vi "10. FGV Error handler.vi"(5 "error in (no error)":errorcluster) -> (14 "Error message":string="ERROR NO IDENTIFICADO", 15 "Error code":i32)   [LabVIEW 2014]
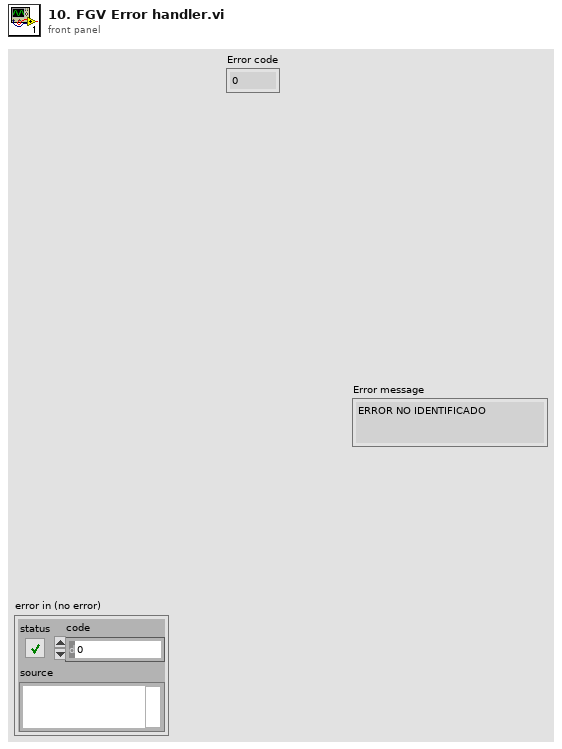
[diagram p1: front panel]
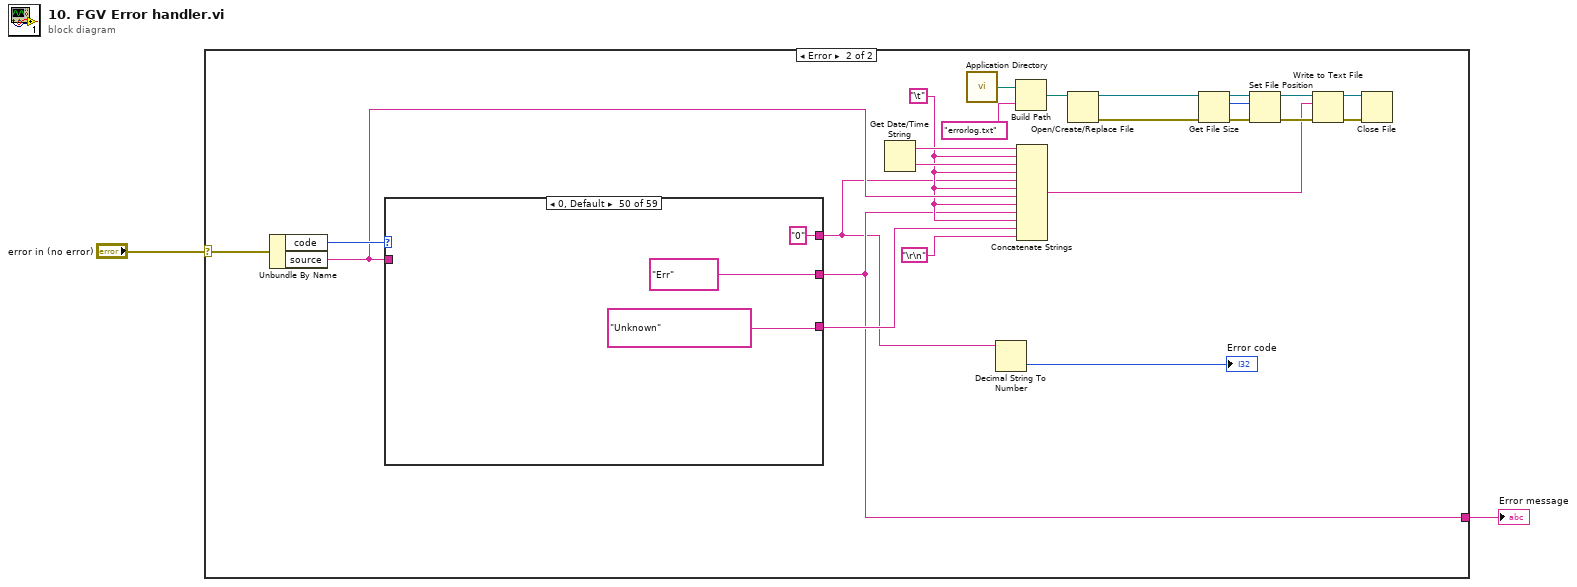
[diagram p0: block diagram]
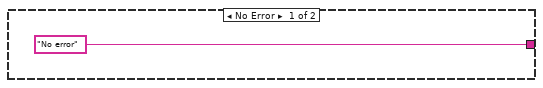
[diagram p2: hidden frame]
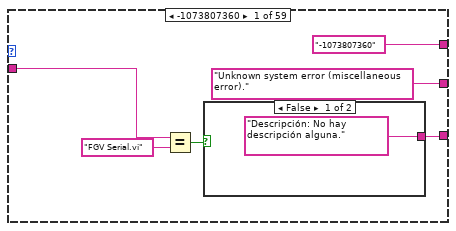
[diagram p3: hidden frame]
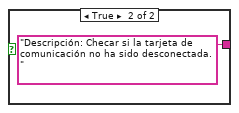
[diagram p4: hidden frame]
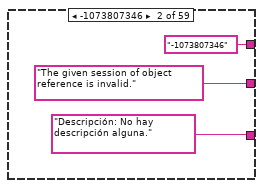
[diagram p5: hidden frame]
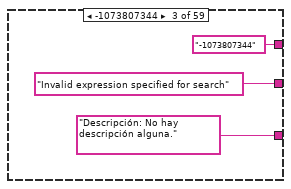
[diagram p6: hidden frame]
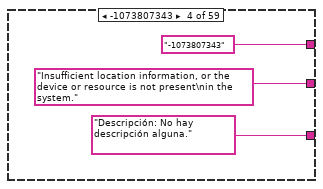
[diagram p7: hidden frame]
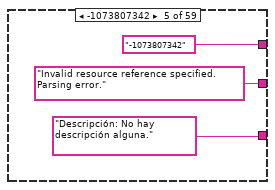
[diagram p8: hidden frame]
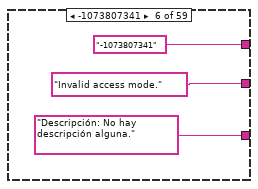
[diagram p9: hidden frame]
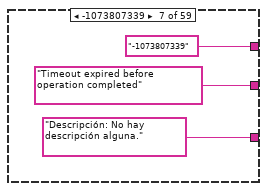
[diagram p10: hidden frame]
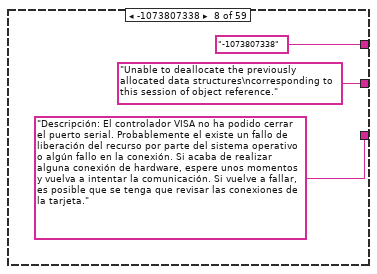
[diagram p11: hidden frame]
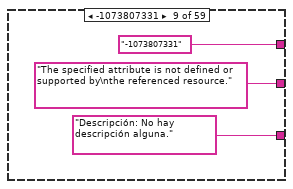
[diagram p12: hidden frame]
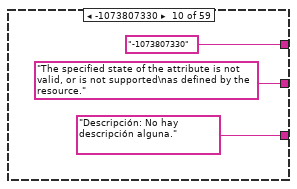
[diagram p13: hidden frame]
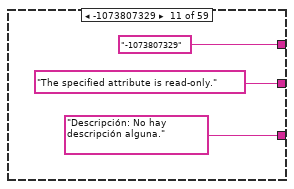
[diagram p14: hidden frame]
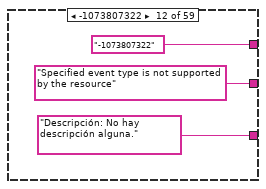
[diagram p15: hidden frame]
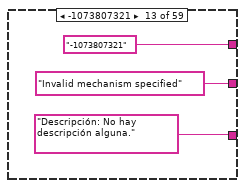
[diagram p16: hidden frame]
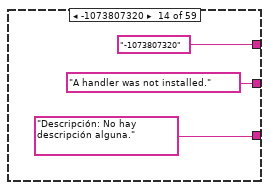
[diagram p17: hidden frame]
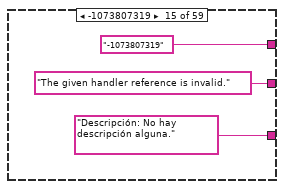
[diagram p18: hidden frame]
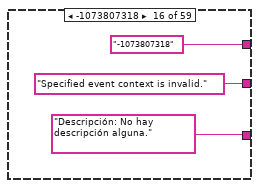
[diagram p19: hidden frame]
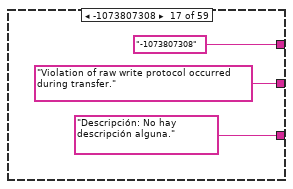
[diagram p20: hidden frame]
diagram:
  n1 = case shown="Error" "error in (no error)" {
    selector: "error in (no error)" -> [_ w26]
    tunnel: ["No error" w6] -> w1
    frame No Error {
    }
    frame Error {
      w9 = "\t"
      n2 = Unbundle By Name(w26) -> ("code"=w27:i32, "source"=w10:string)
      n3 = case shown="0, Default" w27 {
        tunnel: w10 -> [w29 _ _ _ _ _ _ _ _ _ _ _ _ _ _ _ _ _ _ _ _ _ _ _ _ _ _ _ _ _ _ _ _ _ _ _ _ _ _ _ _ _ _ _ _ _ _ _ _ _ _ _ _ _ _ _ _ _ _]
        tunnel: ["Unknown system error (miscellaneous error)." "The given session of object reference is invalid." "Invalid expression specified for search" "Insufficient location information, or the device or resource is not present\nin the system." "Invalid resource reference specified. Parsing error." "Invalid access mode." "Timeout expired before operation completed" "Unable to deallocate the previously allocated data structures\ncorresponding to this session of object reference." "The specified attribute is not defined or supported by\nthe referenced resource." "The specified state of the attribute is not valid, or is not supported\nas defined by the resource." "The specified attribute is read-only." "Specified event type is not supported by the resource" "Invalid mechanism specified" "A handler was not installed." "The given handler reference is invalid." "Specified event context is invalid." "Violation of raw write protocol occurred during transfer." "Violation of raw read protocol occurred during transfer." "Device reported an output protocol error during transfer." "Device reported an input protocol error during transfer." "Bus error occurred during transfer." "Unable to start operation because setup is invalid (due to attributes being set to an inconsistent state)." "Insufficient system resources to perform necessary memory allocation." "Invalid buffer mask specified." "Could not perform read/write operation because of I/O error." "A format specifier in the format string is invalid." "A format specifier in the format string is not supperted." "The specified trigger line is currently in use." "Service request has not been received for the session." "Invalid address space specified." "Invalid offset specified." "Specified offset is not accessible from this hardware." "The specified session is not currently mapped." "No listeners condition is detected (both NRFD and NDAC are deasserted)." "The interface associated with this session is not currently the controller in charge." "The given session or object reference does not support this operation." "Specified width is not supported by this hardware." "The protocol specified is invalid." "Invalid size of window specified." "The specified session already contains a mapped window." "The given operation is not implemented." "User stopped application" "Data bad" "Unrecognized command" "Bad Checksum" "Timeout: EOT not found" "Bad counter" "Timeout: Empty buffer" "Timeout: SOH not found" "Err" "HC16 is busy" "STA Timeout" "STA input timeout" "STA output timeout" "Serial port parity error." "Serial port overrun error." "Serial port receive buffer overflow." "Serial port framing error." "Serial port timeout; bytes not receiveed at serial port"] -> w6
        tunnel: ["-1073807360" "-1073807346" "-1073807344" "-1073807343" "-1073807342" "-1073807341" "-1073807339" "-1073807338" "-1073807331" "-1073807330" "-1073807329" "-1073807322" "-1073807321" "-1073807320" "-1073807319" "-1073807318" "-1073807308" "-1073807307" "-1073807306" "-1073807305" "-1073807304" "-1073807302" "-1073807300" "-1073807299" "-1073807298" "-1073807297" "-1073807295" "-1073807294" "-1073807286" "-1073807282" "-1073807279" "-1073807276" "-1073807273" "-1073807265" "-1073807264" "-1073807257" "-1073807242" "-1073807239" "-1073807237" "-1073807232" "-1073807231" "-8" "-7" "-6" "-5" "-4" "-3" "-2" "-1" "0" "1" "2" "3" "4" "61" "62" "63" "64" "65"] -> w5
        tunnel: [w32 "Descripción: No hay descripción alguna." "Descripción: No hay descripción alguna." "Descripción: No hay descripción alguna." "Descripción: No hay descripción alguna." "Descripción: No hay descripción alguna." "Descripción: No hay descripción alguna." "Descripción: El controlador VISA no ha podido cerrar el puerto serial. Probablemente el existe un fallo de liberación del recurso por parte del sistema operativo o algún fallo en la conexión. Si acaba de realizar alguna conexión de hardware, espere unos momentos y vuelva a intentar la comunicación. Si vuelve a fallar, es posible que se tenga que revisar las conexiones de la tarjeta." "Descripción: No hay descripción alguna." "Descripción: No hay descripción alguna." "Descripción: No hay descripción alguna." "Descripción: No hay descripción alguna." "Descripción: No hay descripción alguna." "Descripción: No hay descripción alguna." "Descripción: No hay descripción alguna." "Descripción: No hay descripción alguna." "Descripción: No hay descripción alguna." "Descripción: No hay descripción alguna." "Descripción: No hay descripción alguna." "Descripción: No hay descripción alguna." "Descripción: No hay descripción alguna." "Descripción: No hay descripción alguna." "Descripción: No hay descripción alguna." "Descripción: No hay descripción alguna." "Descripción: No hay descripción alguna." "Descripción: No hay descripción alguna." "Descripción: No hay descripción alguna." "Descripción: No hay descripción alguna." "Descripción: No hay descripción alguna." "Descripción: No hay descripción alguna." "Descripción: No hay descripción alguna." "Descripción: No hay descripción alguna." "Descripción: No hay descripción alguna." "Descripción: No hay descripción alguna." "Descripción: No hay descripción alguna." "Descripción: No hay descripción alguna." "Descripción: No hay descripción alguna." "Descripción: No hay descripción alguna." "Descripción: No hay descripción alguna." "Descripción: No hay descripción alguna." "Descripción: No hay descripción alguna." "Descripción: El usuario abortó la aplicación y es probable que algunos datos se hayan perdido. Vuelva a iniciar la aplicación." "Descripión: Datos corruptos. Vuelva a intentar la transmisión o realice ajustes en la configuración de conexión." "Descripción: Vuelva a intentar la transmisión." "Descripción: Se han perdido datos durante la recepción. Vuelva a intentar la transmisión." "Descripción: Mensaje incompleto. Intente con un timeout mayor" "Descripción: Vuelva a intentar la transmisión." "Descripción: No hay respuesta de emisor. Ajuste el timeout con valor mayor." "Descripción: Vuelve a intentar con un timeout mayor." "Unknown" "Descripción: La soldadora no puede recibir información por el momento ya sea porque está realizando otra operación o porque el puerto está ocupado." "Descripción: Terminó el tiempo de espera del STA, vuelva a enviar el mensaje." "Descripción: El STA no recibió datos de entrada. Vuelva a intentar la comunicación." "Descripción: El tiempo de espera del STA se acabó, intente de nuevo la comunicación." "Descripción: No hay descripción alguna." "Descripción: No hay descripción alguna." "Descripción: No hay descripción alguna." "Descripción: No hay descripción alguna." "Descripción: No hay descripción alguna."] -> w8
        frame -1073807360 {
          n4 = Equal?(x=w29, y="FGV Serial.vi") -> (x = y?=w30:bool)
          n5 = case shown="False" w30 {
            tunnel: ["Descripción: No hay descripción alguna." "Descripción: Checar si la tarjeta de comunicación no ha sido desconectada."] -> w32
            frame False {
            }
            frame True {
            }
          }
        }
        frame -1073807346 {
        }
        frame -1073807344 {
        }
        frame -1073807343 {
        }
        frame -1073807342 {
        }
        frame -1073807341 {
        }
        frame -1073807339 {
        }
        frame -1073807338 {
        }
        frame -1073807331 {
        }
        frame -1073807330 {
        }
        frame -1073807329 {
        }
        frame -1073807322 {
        }
        frame -1073807321 {
        }
        frame -1073807320 {
        }
        frame -1073807319 {
        }
        frame -1073807318 {
        }
        frame -1073807308 {
        }
        frame -1073807307 {
        }
        frame -1073807306 {
        }
        frame -1073807305 {
        }
        frame -1073807304 {
        }
        frame -1073807302 {
        }
        frame -1073807300 {
        }
        frame -1073807299 {
        }
        frame -1073807298 {
        }
        frame -1073807297 {
        }
        frame -1073807295 {
        }
        frame -1073807294 {
        }
        frame -1073807286 {
        }
        frame -1073807282 {
        }
        frame -1073807279 {
        }
        frame -1073807276 {
        }
        frame -1073807273 {
        }
        frame -1073807265 {
        }
        frame -1073807264 {
        }
        frame -1073807257 {
        }
        frame -1073807242 {
        }
        frame -1073807239 {
        }
        frame -1073807237 {
        }
        frame -1073807232 {
        }
        frame -1073807231 {
        }
        frame -8 {
        }
        frame -7 {
        }
        frame -6 {
        }
        frame -5 {
        }
        frame -4 {
        }
        frame -3 {
        }
        frame -2 {
        }
        frame -1 {
        }
        frame 0, Default {
        }
        frame 1 {
        }
        frame 2 {
        }
        frame 3 {
        }
        frame 4 {
        }
        frame 61 {
        }
        frame 62 {
        }
        frame 63 {
        }
        frame 64 {
        }
        frame 65 {
        }
      }
      n6 = Get Date/Time String() -> (date string=w11:string, time string=w12:string)  [unwired: 3 in]
      n7 = call <vilib>:"Application Directory.vi"() -> ("Application Directory"=w24:path)
      n8 = Decimal String To Number(string=w5) -> (number=→"Error code":i32)  [unwired: 2 in, 1 out]
      n9 = Build Path(base path=w24, name or relative path="errorlog.txt") -> (appended path=w25:path)
      n10 = Concatenate Strings(w11, w9, w12, w9, w5, w9, w10, w9, w6, w9, w8, "\r\n") -> (w13:string)
      n11 = Open/Create/Replace File(file path (use dialog)=w25) -> (refnum out=w17:refnum<file>, error out=w18:errorcluster)  [unwired: 5 in, 1 out]
      n12 = Get File Size(file=w17, error in=w18) -> (refnum out=w16:refnum<file>, size (in bytes)=w15:i64, 0:w19:errorcluster)
      n13 = Set File Position(offset (in bytes) (0)=w15, refnum=w16, error in=w19) -> (refnum out=w14:refnum<file>, error out=w20:errorcluster)  [unwired: 1 in]
      n14 = Write to Text File(file (use dialog)=w14, text=w13, error in=w20) -> (refnum out=w22:refnum<file>, error out=w21:errorcluster)  [unwired: 1 in, 1 out]
      n15 = Close File(refnum=w22, error in=w21) -> ()  [unwired: 2 out]
    }
  }
  "Error message" <- w1
